vi "Insert SubVI.vi"(4 "Value 2":variant, 5 "Value 1":variant, 6 "Label 2":string, 7 "Label 1":string, 8 "error in (no error)":errorcluster, 10 "VI Path":path) -> (0 "error out":errorcluster, 2 "vi reference":refnum<vi>)   [LabVIEW 2020, in "3D Plot.lvclass"]
uses:
  3D Plot.lvclass
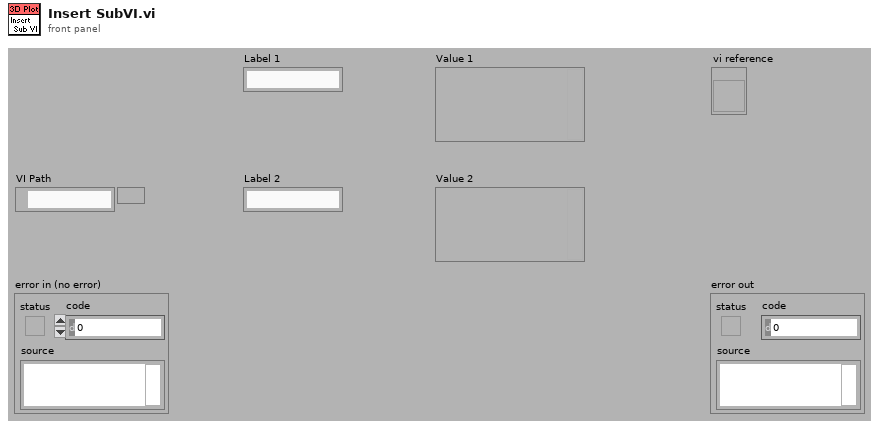
[diagram p1: front panel]
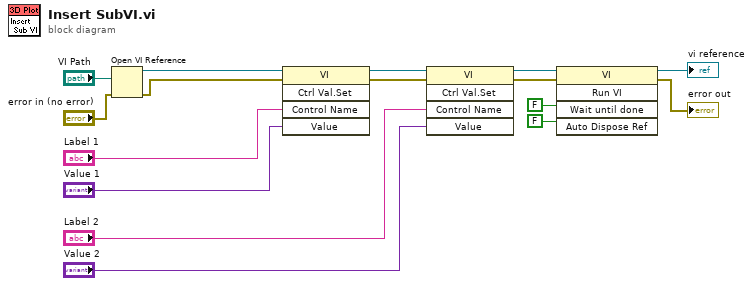
[diagram p0: block diagram]
diagram:
  n1 = Open VI Reference(vi path="VI Path", error in (no error)="error in (no error)") -> (vi reference=w9:refnum<vi>, error out=w1:errorcluster)  [unwired: 1 in, 3 out]
  n2 = invoke class="VI" method="Ctrl Val.Set"(reference=w9, error in=w1, "Control Name"="Label 1", "Value"="Value 1") -> (reference out=w12:refnum<vi>, error out=w16:errorcluster)  [unwired: 1 in, 3 out]
  n3 = invoke class="VI" method="Ctrl Val.Set"(reference=w12, error in=w16, "Control Name"="Label 2", "Value"="Value 2") -> (reference out=w13:refnum<vi>, error out=w14:errorcluster)  [unwired: 1 in, 3 out]
  n4 = invoke class="VI" method="Run VI"(reference=w13, error in=w14, "Wait until done"=FALSE ("Wait Until Done"), "Auto Dispose Ref"=FALSE ("Auto Dispose Reference")) -> (reference out=→"vi reference":refnum<vi>, error out=→"error out":errorcluster)  [unwired: 1 in, 3 out]
